vi "2-2.vi"(6 "kf(Hz/V)":dbl=50000.0, 8 "An(V)":dbl=0.1, 9 "带通Butterworth滤波器":cluster{"中心频率(Hz)":dbl, "带宽(Hz)":dbl}={"中心频率(Hz)"=150000.0, "带宽(Hz)"=280000.0}, 10 "调制信号":T1={"fm1(Hz)"=5000.0, "Am(V)"=1.0, "fm2(Hz)"=3000.0}, 11 "载波信号":cluster{"fc(Hz)":dbl, "Ac(V)":dbl}={"fc(Hz)"=150000.0, "Ac(V)"=1.0}) -> (1 "频域":cluster{"f0":dbl, "df":dbl, "magnitude":dbl[]}(graph), 2 "时域 2":waveform(dbl)[](graph), 3 "时域":waveform(dbl)[](graph))   [LabVIEW 2018]
uses:
  <vilib>/Analysis/3filter.llb/Filter Passband Type.ctl
  <vilib>/Analysis/3filter.llb/Butterworth Filter (DBL).vi
  <vilib>/express/express analysis/Spectral/Block/exnSpectralBlock spectral measurements peak poly.vi
  <vilib>/express/express analysis/Spectral/Block/exnSpectralBlock spectral measurements peak WFM.vi
  <vilib>/express/express analysis/Spectral/XNode/ExpressSpectralMeasurementsBlockNode.xnode
  <vilib>/measure/NI_MABase.lvlib
  <vilib>/Analysis/NI_AALPro.lvlib
  <vilib>/Analysis/NI_AALBase.lvlib
panel:
  out "BT（卡森定则）":dbl[](array[numeric])
  out "fm2成分":waveform(dbl)(graph)
  out "fh":dbl
  out "fl":dbl
  in  "选项卡控件":enum32{"调制", "滤波", "解调"}(tab)
  out "频域":cluster{"f0":dbl, "df":dbl, "magnitude":dbl[]}(graph)
  out "时域":waveform(dbl)(graph)
  out "数组":dbl[](array[numeric])
  out "fm1成分":waveform(dbl)(graph)
  out "积分信号":waveform(dbl)(graph)
  out "采样参数（采样频率fs，采样数Ns）":cluster{dbl, dbl} {"?" format="%#_6f"; "?" format="%#_6f"}
  out "载波信号":waveform(dbl)(graph)
  # "要显示n个周期的调制信号波形，\n则采样数Ns=n*fs/fm\nfh和fl为滤波器实际取的参数"
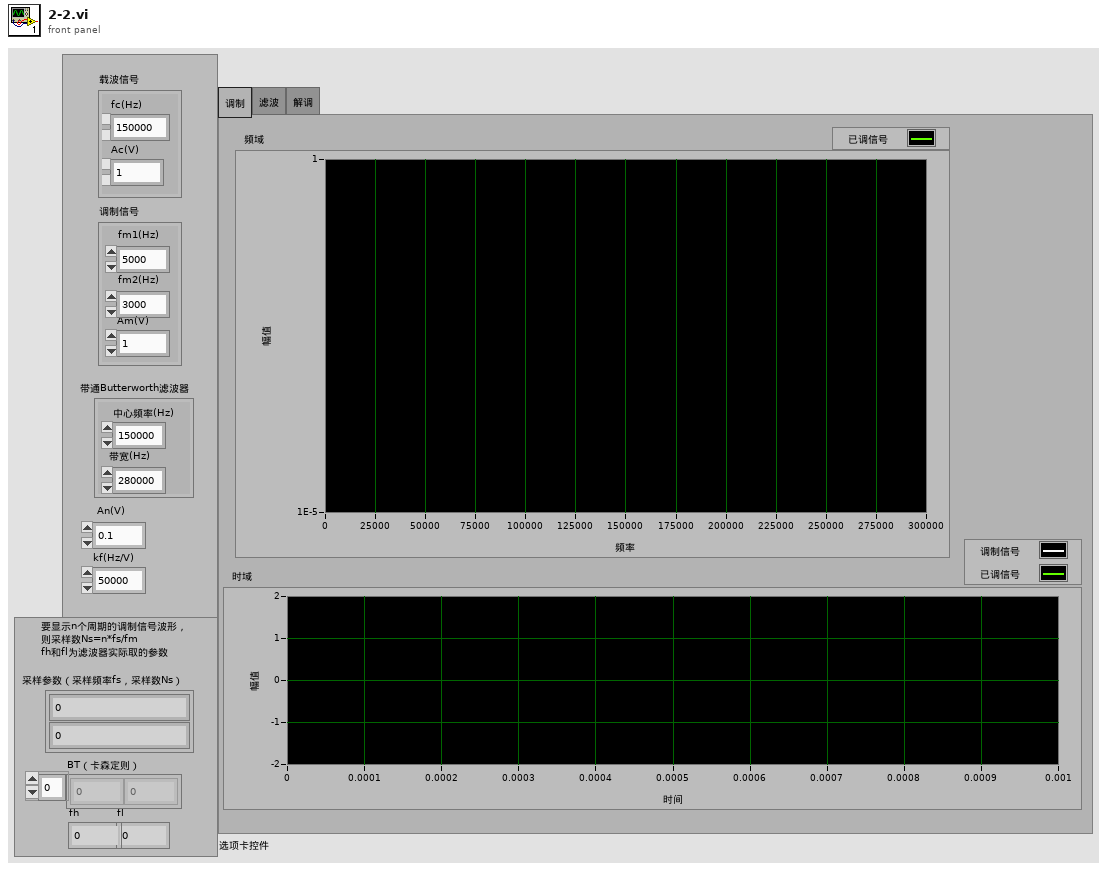
[diagram p1: front panel]
types:
  T1 = cluster{"fm1(Hz)":dbl, "Am(V)":dbl, "fm2(Hz)":dbl}
  T2 = typedef "NI_AALBase.lvlib/Filter Passband Type.ctl" = enum32{"Lowpass", "Highpass", "Bandpass", "Bandstop"}
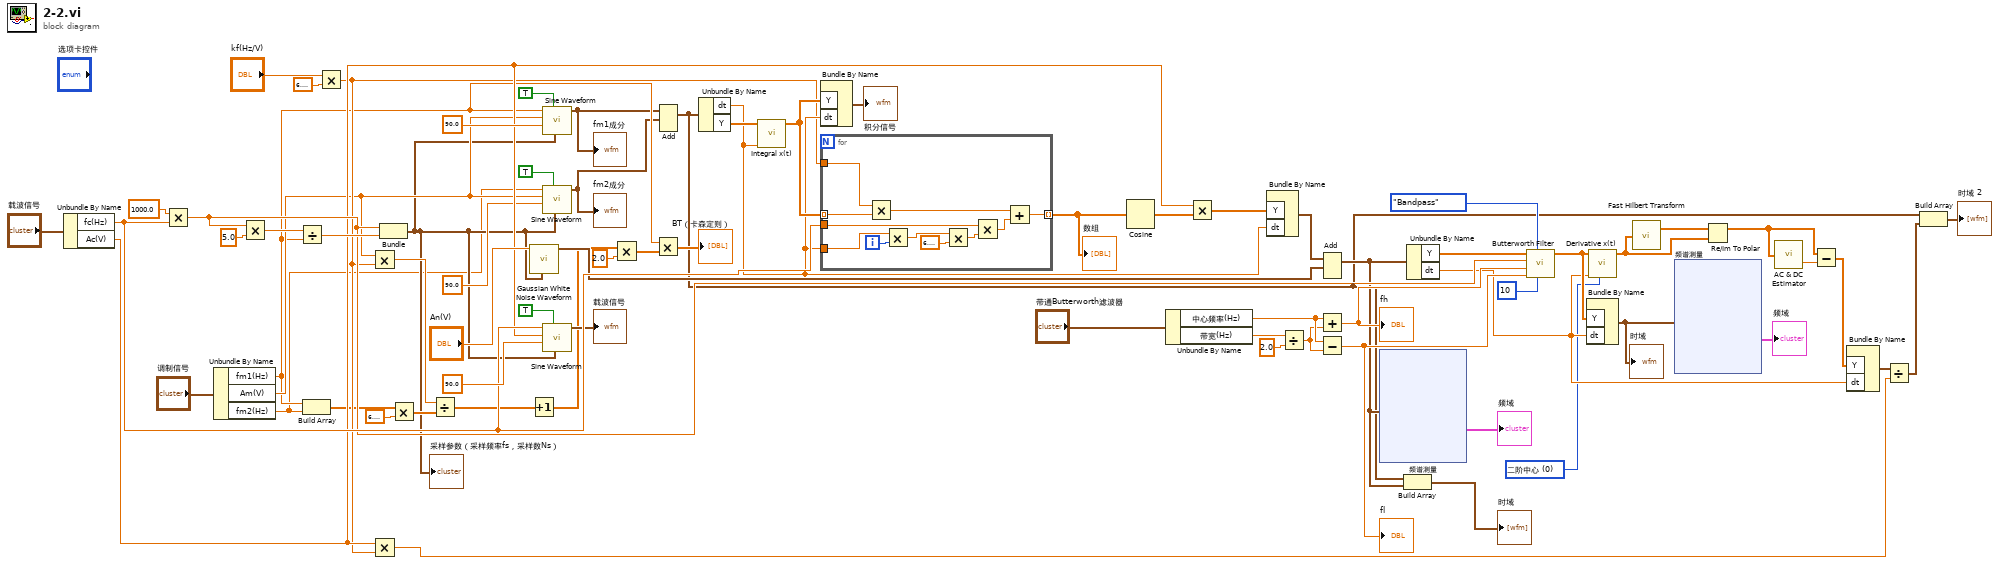
[diagram p0: block diagram]
diagram:
  w24 = u16 0 items=["二阶中心", "四阶中心", "前向", "后向"] ("method")
  n1 = Unbundle By Name("载波信号") -> ("fc(Hz)"=w59:dbl, "Ac(V)"=w20:dbl)
  n2 = Multiply(x=1000.0, y=w59) -> (x*y=w32:dbl)
  n3 = Unbundle By Name("调制信号") -> ("fm1(Hz)"=w7:dbl, "Am(V)"=w9:dbl, "fm2(Hz)"=w6:dbl)
  n4 = Multiply(x=w32, y=5.0) -> (x*y=w67:dbl)
  n5 = Divide(x=w67, y=w7) -> (x/y=w66:dbl)
  n6 = Build Array(w7, w6) -> (w5:dbl[])
  n7 = Multiply(x="kf(Hz/V)", y=6.283185307179586) -> (x*y=w14:dbl)
  n8 = Multiply(x=w9, y=w14) -> (x*y=w46:dbl)
  n9 = Multiply(x=w20, y=w14) -> (x*y=w18:dbl)
  n10 = Bundle(w32, w66) -> (w8:cluster{dbl, dbl})  [unwired: 1 in]
  "采样参数（采样频率fs，采样数Ns）" <- w8
  n11 = Multiply(x=w5, y=6.283185307179586) -> (x*y=w47:dbl[])
  n12 = Divide(x=w46, y=w47) -> (x/y=w45:dbl[])
  n13 = call <vilib>:"Gaussian White Noise Waveform.vi"("sampling info"=w8, "standard deviation"="An(V)") -> ("signal out"=w51:waveform(dbl))  [unwired: 8 in, 1 out]
  n14 = Increment(x=w45) -> (x+1=w44:dbl[])
  n15 = call <vilib>:"Sine Waveform.vi"("sampling info"=w8, "reset signal"=TRUE, "phase"=90.0, "amplitude"=w9, "frequency"=w7) -> ("signal out"=w2:waveform(dbl))  [unwired: 5 in, 1 out]
  "fm1成分" <- w2
  n16 = call <vilib>:"Sine Waveform.vi"("sampling info"=w8, "reset signal"=TRUE, "phase"=90.0, "amplitude"=w9, "frequency"=w6) -> ("signal out"=w3:waveform(dbl))  [unwired: 5 in, 1 out]
  "fm2成分" <- w3
  n17 = call <vilib>:"Sine Waveform.vi"("sampling info"=w8, "reset signal"=TRUE, "phase"=90.0, "amplitude"=w20, "frequency"=w59) -> ("signal out"=→"载波信号":waveform(dbl))  [unwired: 5 in, 1 out]
  n18 = Multiply(x=w44, y=2.0) -> (x*y=w42:dbl[])
  n19 = Add(1:w3, 2:w2) -> (0:w1:waveform(dbl))  [unwired: 1 in, 1 out]
  n20 = Multiply(x=w7, y=w42) -> (x*y=→"BT（卡森定则）":dbl[])
  n21 = Unbundle By Name(w1) -> ("dt"=w56:dbl, "Y"=w68:dbl[])
  n22 = call <vilib>:"Integral x(t).vi"("dt"=w56, "X"=w68) -> ("Integral X"=w60:dbl[])  [unwired: 8 in, 1 out]
  n23 = Bundle By Name("Y"=w60, "dt"=w56) -> (→"积分信号":waveform(dbl))  [unwired: 1 in]
  n24 = for {
    tunnel: w60 -> [w83] mode=indexing
    tunnel: w56 -> [w81]
    tunnel: w59 -> [w77]
    tunnel: [w74] -> w58 mode=indexing
    tunnel: w14 -> [w73]
    i -> [w82]
    n25 = Multiply(x=w73, y=w83) -> (x*y=w75:dbl)
    n26 = Multiply(x=w81, y=w82) -> (x*y=w79:dbl)
    n27 = Multiply(x=w79, y=6.283185307179586) -> (x*y=w78:dbl)
    n28 = Multiply(x=w77, y=w78) -> (x*y=w76:dbl)
    n29 = Add(x=w75, y=w76) -> (x+y=w74:dbl)
  }
  "数组" <- w58
  n30 = Cosine(x=w58) -> (cos(x)=w57:dbl[])
  n31 = Unbundle By Name("带通Butterworth滤波器") -> ("中心频率(Hz)"=w34:dbl, "带宽(Hz)"=w38:dbl)
  n32 = Multiply(x=w20, y=w57) -> (x*y=w55:dbl[])
  n33 = Bundle By Name("Y"=w55, "dt"=w56) -> (w53:waveform(dbl))  [unwired: 1 in]
  n34 = Divide(x=w38, y=2.0) -> (x/y=w33:dbl)
  n35 = Add(1:w51, 2:w53) -> (0:w30:waveform(dbl))  [unwired: 1 in, 1 out]
  n36 = Add(x=w34, y=w33) -> (x+y=w36:dbl)
  "fh" <- w36
  n37 = Subtract(x=w34, y=w33) -> (x-y=w35:dbl)
  "fl" <- w35
  n38 = xnode "频谱测量"("信号"=w30) -> ("FFT - （峰值）"=→"频域":cluster{"f0":dbl, "df":dbl, "magnitude":dbl[]})  [unwired: 1 in, 2 out]
  n39 = Build Array(w1, w30) -> (→"时域":waveform(dbl)[])
  n40 = Unbundle By Name(w30) -> ("Y"=w29:dbl[], "dt"=w25:dbl)
  n41 = call-poly <vilib>:"Butterworth Filter.vi"("order"=10, "filter type"=Filter_Passband_Type."Bandpass", "low cutoff freq: fl"=w35, "high cutoff freq: fh"=w36, "sampling freq: fs"=w32, "X"=w29) -> ("Filtered X"=w27:dbl[])  [unwired: 2 in, 1 out]
  n42 = Bundle By Name("Y"=w27, "dt"=w25) -> (w28:waveform(dbl))  [unwired: 1 in]
  "时域" <- w28
  n43 = call <vilib>:"Derivative x(t).vi"("method"=w24, "dt"=w25, "X"=w27) -> ("dX/dt"=w17:dbl[])  [unwired: 7 in, 1 out]
  n44 = call <vilib>:"Fast Hilbert Transform.vi"("X"=w17) -> ("Hilbert{X}"=w26:dbl[])  [unwired: 1 out]
  n45 = xnode "频谱测量"("信号"=w28) -> ("FFT - （峰值）"=→"频域":cluster{"f0":dbl, "df":dbl, "magnitude":dbl[]})  [unwired: 1 in, 2 out]
  n46 = Re/Im To Polar(2:w17, 3:w26) -> (1:w23:dbl[])  [unwired: 1 out]
  n47 = call <vilib>:"AC & DC Estimator.vi"("Signal (V)"=w23) -> ("DC estimate (V)"=w22:dbl)  [unwired: 1 out]
  n48 = Subtract(x=w23, y=w22) -> (x-y=w21:dbl[])
  n49 = Bundle By Name("Y"=w21, "dt"=w25) -> (w19:waveform(dbl))  [unwired: 1 in]
  n50 = Divide(x=w19, y=w18) -> (x/y=w13:waveform(dbl))
  n51 = Build Array(w1, w13) -> (→"时域 2":waveform(dbl)[])
